vi "DIO.vi"() -> ()   [LabVIEW 2016]
panel:
  in  "DO":bool[](array[boolean])
  out "DI":bool[](array[boolean])
  out "error out":errorcluster caption="错误输出"
  in  "停止":bool
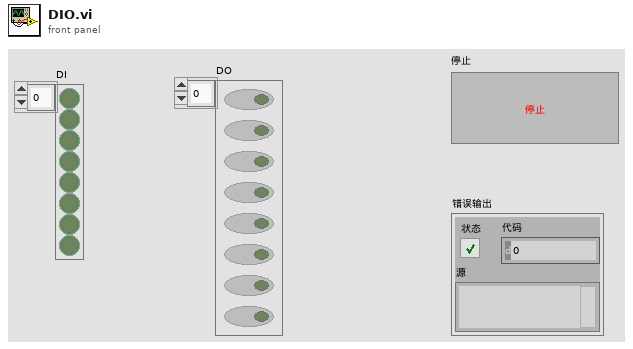
[diagram p1: front panel]
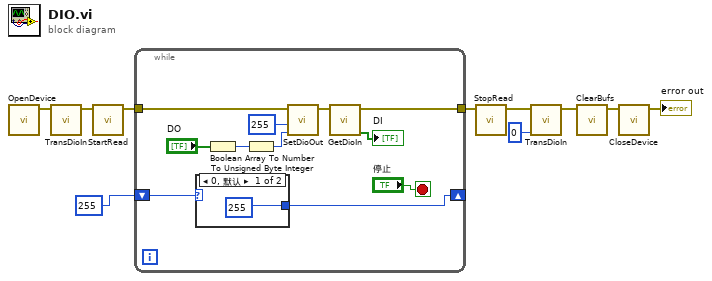
[diagram p0: block diagram]
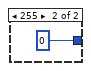
[diagram p2: hidden frame]
diagram:
  n1 = call "OpenDevice.vi"() -> ("error out"=w7:errorcluster)  [unwired: 11 in]
  n2 = call "TransDioIn.vi"("error in"=w7) -> ("error out"=w6:errorcluster)  [unwired: 10 in]
  n3 = call "StartRead.vi"("error in"=w6) -> ("error out"=w10:errorcluster)  [unwired: 10 in]
  n4 = while {
    tunnel: w10 -> [w20]
    tunnel: [w17] -> w5
    shift-right: [w13] -> _
    shift-left: u8 255 ("DioChanSel") -> [w12]
    stop <- "停止" stop-if-true
    n5 = case shown="0, 默认" w12 {
      tunnel: [u8 255 ("DioChanSel") u8 0 ("DioChanSel")] -> w13
      frame 0, Default {
      }
      frame 255 {
      }
    }
    n6 = Boolean Array To Number(Boolean array="DO") -> (number=w14:u32)
    n7 = To Unsigned Byte Integer(number=w14) -> (unsigned 8bit integer=w11:u8)
    n8 = call "SetDioOut.vi"("DioOut"=w11, "DioChanSel"=u8 255, "error in"=w20) -> ("error out"=w19:errorcluster)  [unwired: 8 in]
    n9 = call "GetDioIn.vi"("error in"=w19) -> ("DIO"=→"DI":bool[], "error out"=w17:errorcluster)  [unwired: 8 in, 1 out]
  }
  n10 = call "StopRead.vi"("error in"=w5) -> ("error out"=w4:errorcluster)  [unwired: 10 in]
  n11 = call "TransDioIn.vi"("TransDioInSwitch"=u8 0, "error in"=w4) -> ("error out"=w2:errorcluster)  [unwired: 9 in]
  n12 = call "ClearBufs.vi"("error in"=w2) -> ("error out"=w9:errorcluster)  [unwired: 10 in]
  n13 = call "CloseDevice.vi"("error in"=w9) -> ("error out"=→"error out":errorcluster)  [unwired: 10 in]
